vi "StimFile (G3)-Compute Max Level.vi"(0 "File":T5, 1 "Destination":string, 5 "Filter":T3 {"Stages"."IIR Filter"."Forward Coefficients" format="%.4f"; "Stages"."IIR Filter"."Reverse Coefficients" format="%.4f"}, 9 "Level":T1, 11 "error in (no error)":errorcluster, 12 "Sampling Rate (Hz)":dbl, 13 "Npts":i32) -> (6 "Max Level":dbl, 10 "Level out":T1, 15 "error out":errorcluster)   [LabVIEW 2020]
uses:
  Waveform VIs/File VIs/StimFile-Params.ctl
  Controls/Advanced Filter XCtl/Filter Data.ctl
  Filter VIs/Filter-Bandwidth Units.ctl
  XControls/Level (G3)/Level Data.ctl
  XControls/Level (G3)/Level Units (G3).ctl
  <vilib>/Analysis/5stat.llb/RMS (DBL).vi
  PXI DAQ VIs/DAQ Engine VIs/PXI Globals.vi
  Utility VIs/Math VIs/Linear to dB (scalar).vi
  <vilib>/Analysis/NI_AALPro.lvlib
  <vilib>/Analysis/2dsp.llb/Inverse Complex FFT.vi
  Controls/Advanced Filter XCtl/Advanced Filter XCtl.xctl
  XControls/Level (G3)/Level (G3).xctl
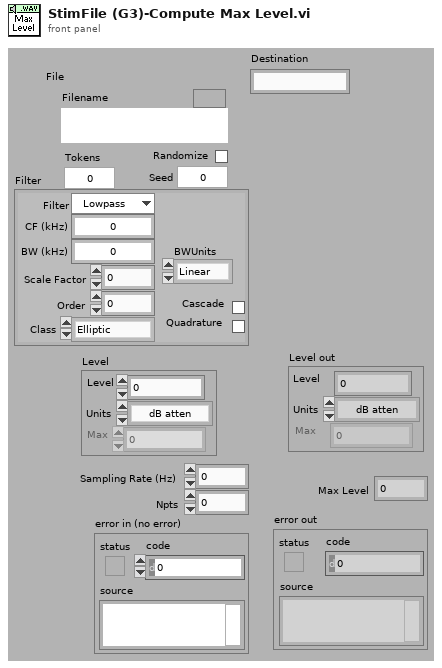
[diagram p1: front panel]
types:
  T1 = typedef "Level (G3).xctl/Level Data.ctl" = cluster{"Level":dbl, "Units":T2, "Max":dbl, "Data":cluster{"Multiplier":dbl, "Cal File":path, "Cal":cluster{"Freq (Hz)":dbl[], "Mag (dB SPL)":dbl[], "Phase (deg)":dbl[]}, "audiogram":path}}
  T2 = typedef "Level (G3).xctl/Level Units (G3).ctl" = enum16{"dB atten", "dB SPL", "dB re 1 Vrms", "dB V/Hz½", "mW", "dB HL", "Volts", "dB mW"}
  T3 = typedef "Advanced Filter XCtl.xctl/Filter Data.ctl" = cluster{"Type":enum16{"Lowpass", "Highpass", "Bandpass", "Bandstop", "OFF"}, "CF (kHz)":dbl, "BW (kHz)":dbl, "Cascade":bool, "Quadrature":bool, "Scale Factor":dbl, "Stages":cluster{"IIR Filter":cluster{"filter structure":enum32{"IIR 2nd Order", "IIR 4th Order"}, "Reverse Coefficients":dbl[], "Forward Coefficients":dbl[]}, "State":dbl[]}[], "Class":enum16{"Elliptic", "Butterworth"}, "Order":i32, "BWUnits":T4}
  T4 = typedef "Filter-Bandwidth Units.ctl" = enum16{"Linear", "Octaves", "Min-Max"}
  T5 = typedef "StimFile-Params.ctl" = cluster{"Filename":path, "Signal":dbl[], "Channel":i32, "stream":bool, "offset":i32, "nreps":i32, "loops":i32, "Randomize":bool, "order":i32[], "Seed":i32, "Tokens":i32}
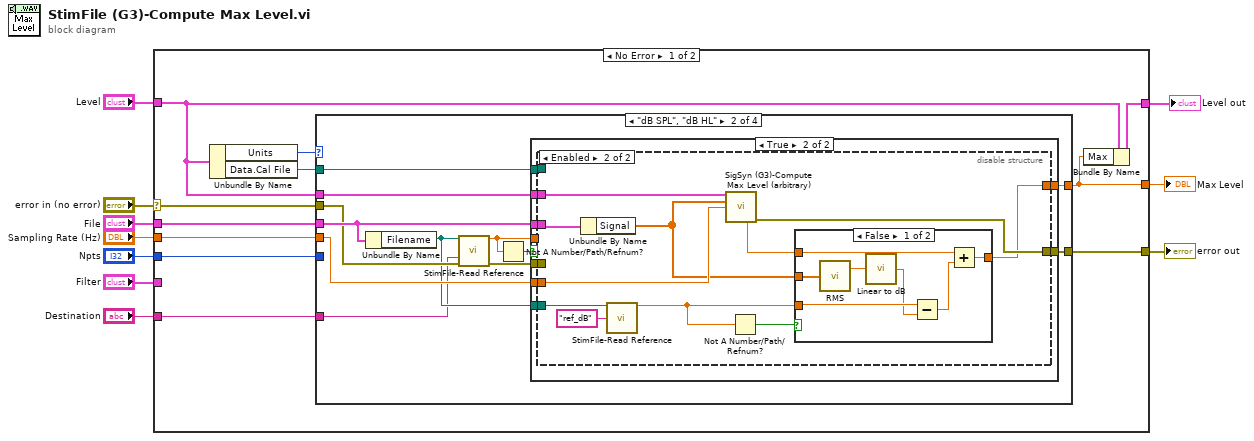
[diagram p0: block diagram]
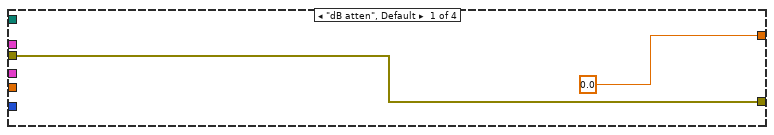
[diagram p2: hidden frame]
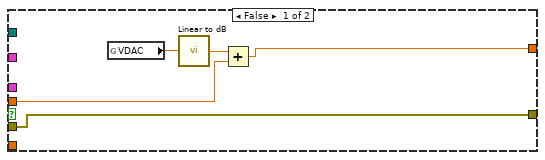
[diagram p3: hidden frame]
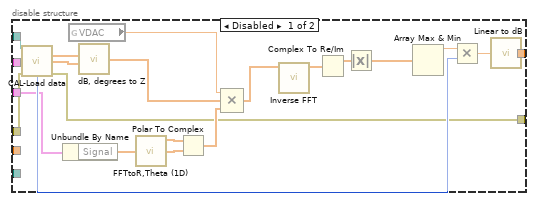
[diagram p4: hidden frame]
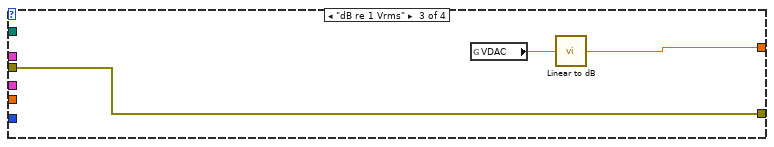
[diagram p6: hidden frame]
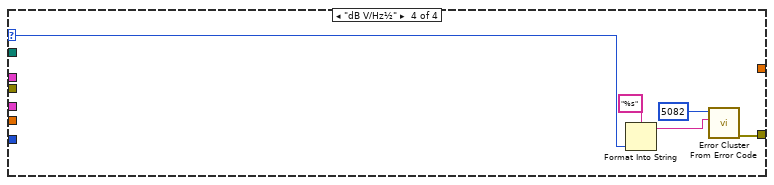
[diagram p7: hidden frame]
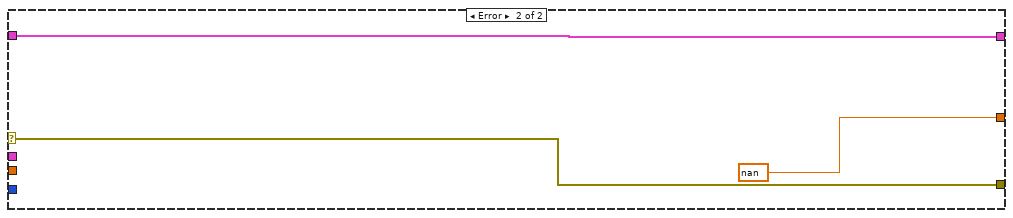
[diagram p8: hidden frame]
diagram:
  n1 = case shown="No Error" "error in (no error)" {
    selector: "error in (no error)" -> [w21 w98]
    tunnel: "Level" -> [w12 w96]
    tunnel: "File" -> [w13 _]
    tunnel: "Filter" -> [_ _]
    tunnel: [w18 w98] -> w9
    tunnel: "Npts" -> [w20 _]
    tunnel: [w17 nan ("Reference Level")] -> w4
    tunnel: "Sampling Rate (Hz)" -> [w19 _]
    tunnel: [w16 w96] -> w2
    tunnel: "Destination" -> [w11 _]
    frame No Error {
      n2 = Unbundle By Name(w12) -> ("Units"=w15:T2, "Data.Cal File"=w14:path)
      n3 = case shown="\"dB SPL\", \"dB HL\"" w15 {
        selector: w15 -> [_ _ _ w91]
        tunnel: w21 -> [w22 w31 w88 _]
        tunnel: w20 -> [_ _ _ _]
        tunnel: [0.0 ("Reference Level") w34 w89 _] -> w17
        tunnel: w19 -> [_ w27 _ _]
        tunnel: [w22 w33 w88 w92] -> w18
        tunnel: w14 -> [_ w35 _ _]
        tunnel: w13 -> [_ w32 _ _]
        tunnel: w12 -> [_ w26 _ _]
        tunnel: w11 -> [_ w24 _ _]
        frame "dB atten", Default {
        }
        frame "dB SPL", "dB HL" {
          n4 = Unbundle By Name(w32) -> ("Filename"=w25:path)
          n5 = call "StimFile-Read Reference.vi"("Wave File"=w25, "Destination"=w24, "error in (no error)"=w31) -> ("Reference (dB)"=w28:dbl, "error out"=w30:errorcluster)  [unwired: 10 in, 1 out]
          n6 = Not A Number/Path/Refnum?(number/path/refnum=w28) -> (NaN/Path/Refnum?=w29:bool)
          n7 = case shown="True" w29 {
            tunnel: w30 -> [w40 w48]
            tunnel: w35 -> [_ w47]
            tunnel: [w36 w46] -> w34
            tunnel: [w40 w42] -> w33
            tunnel: w32 -> [_ w45]
            tunnel: w28 -> [w37 _]
            tunnel: w27 -> [_ w44]
            tunnel: w26 -> [_ w43]
            tunnel: w25 -> [_ w41]
            frame False {
              n8 = global read "PXI Globals.vi" "VDAC"() -> (w39:dbl)
              n9 = call-poly "Linear to dB.vi"("Linear"=w39) -> ("dB"=w38:dbl)
              n10 = Add(x=w38, y=w37) -> (x+y=w36:dbl)
            }
            frame True {
              n11 = disable-structure shown="Enabled" {
                disable-tunnel: w48 -> [w68 _]
                disable-tunnel: w47 -> [w67 _]
                disable-tunnel: [w52 w72] -> w46
                disable-tunnel: w45 -> [w50 w79]
                disable-tunnel: w44 -> [_ w78]
                disable-tunnel: w43 -> [_ w77]
                disable-tunnel: [w51 w76] -> w42
                disable-tunnel: w41 -> [_ w75]
                frame Disabled {
                  n12 = call "CAL-Load data.vi"("user path"=w67, "error in (no error)"=w68) -> ("Mag"=w66:dbl[], "Phase"=w65:dbl[], "npts"=w54:i32, "error out"=w51:errorcluster)  [unwired: 6 in, 4 out]
                  n13 = Unbundle By Name(w50) -> ("Signal"=w49:dbl[])
                  n14 = global read "PXI Globals.vi" "VDAC"() -> (w63:dbl)
                  n15 = call "dB, degrees to Z.vi"("Magnitude (dB)"=w66, "Phase (degrees)"=w65) -> ("Z"=w64:cdb[])  [unwired: 5 in]
                  n16 = call "FFTtoR,Theta (1D).VI"("X"=w49) -> ("+Freq. Mag of FFT"=w61:dbl[], "+Freq Theta of FFT"=w62:dbl[])  [unwired: 1 in]
                  n17 = Polar To Complex(1:w62, 2:w61) -> (0:w60:cdb[])
                  n18 = Compound Arithmetic op=MULTIPLY(w63, w64, w60) -> (w59:cdb[])
                  n19 = call-poly <vilib>:"Inverse FFT.vi"("FFT {X}"=w59) -> ("X"=w58:cdb[])  [unwired: 9 in, 1 out]
                  n20 = Complex To Re/Im(x + iy=w58) -> (x=w57:dbl[])  [unwired: 1 out]
                  n21 = Absolute Value(x=w57) -> (abs(x)=w55:dbl[])
                  n22 = Array Max & Min(array=w55) -> (max value=w56:dbl)  [unwired: 3 out]
                  n23 = Multiply(x=w56, y=w54) -> (x*y=w53:dbl)
                  n24 = call-poly "Linear to dB.vi"("Linear"=w53) -> ("dB"=w52:dbl)
                }
                frame Enabled {
                  n25 = Unbundle By Name(w79) -> ("Signal"=w69:dbl[])
                  n26 = call "StimFile-Read Reference.vi"("Wave File"=w75, "refUnits"="ref_dB") -> ("Reference (dB)"=w70:dbl)  [unwired: 11 in, 2 out]
                  n27 = call "SigSyn (G3)-Compute Max Level (arbitrary).vi"("Level"=w77, "Y"=w69, "Sampling Rate (Hz)"=w78) -> ("Max Level"=w71:dbl, "error out"=w76:errorcluster)  [unwired: 10 in, 1 out]
                  n28 = Not A Number/Path/Refnum?(number/path/refnum=w70) -> (NaN/Path/Refnum?=w73:bool)
                  n29 = case shown="False" w73 {
                    tunnel: [w82 w87] -> w72
                    tunnel: w71 -> [w81 w87]
                    tunnel: w70 -> [w84 _]
                    tunnel: w69 -> [w86 _]
                    frame False {
                      n30 = call-poly <vilib>:"RMS.vi"("X"=w86) -> ("rms value"=w85:dbl)  [unwired: 1 out]
                      n31 = call-poly "Linear to dB.vi"("Linear"=w85) -> ("dB"=w83:dbl)
                      n32 = Subtract(x=w84, y=w83) -> (x-y=w80:dbl)
                      n33 = Add(x=w81, y=w80) -> (x+y=w82:dbl)
                    }
                    frame True {
                    }
                  }
                }
              }
            }
          }
        }
        frame "dB re 1 Vrms" {
          n34 = global read "PXI Globals.vi" "VDAC"() -> (w90:dbl)
          n35 = call-poly "Linear to dB.vi"("Linear"=w90) -> ("dB"=w89:dbl)
        }
        frame "dB V/Hz½" {
          n36 = Format Into String(format string="%s", w91) -> (resulting string=w94:string)  [unwired: 2 in, 1 out]
          n37 = call <vilib>:"Error Cluster From Error Code.vi"("error message (\"\")"=w94, "error code (0)"=5082) -> ("error out"=w92:errorcluster)  [unwired: 7 in]
        }
      }
      n38 = Bundle By Name(cluster=w12, "Max"=w17) -> (w16:T1)
    }
    frame Error {
    }
  }
  "error out" <- w9
  "Max Level" <- w4
  "Level out" <- w2
